vi "Eurotherm - Address String.vi"(7 "Address":T1=1 min=1 max=99) -> (8 "String":string)   [LabVIEW 2011]
uses:
  Eurotherm - Controls/Eurotherm - Address.ctl
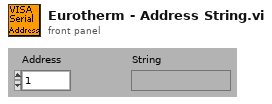
[diagram p1: front panel]
types:
  T1 = typedef "Eurotherm - Address.ctl" = u8
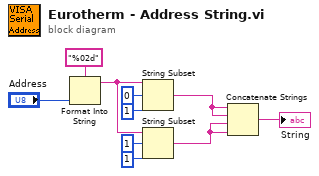
[diagram p0: block diagram]
diagram:
  n1 = Format Into String(format string="%02d", "Address") -> (resulting string=w4:string)  [unwired: 2 in, 1 out]
  n2 = String Subset(string=w4, offset (0)=0, length (rest)=1 ("length (rest)")) -> (substring=w3:string)
  n3 = String Subset(string=w4, offset (0)=1, length (rest)=1 ("length (rest)")) -> (substring=w2:string)
  n4 = Concatenate Strings(w3, w3, w2, w2) -> (→"String":string)
